vi "SaveRestore_Turret_Homing_Calibration.vi"(2 "ReadWrite_Mode":T1, 3 "Turret_Offset (SensorUnits)":i32) -> (0 "Turret_Home_Set":i32, 1 "Load/Save_successful?":bool)   [LabVIEW 2019]
uses:
  TypeDefs/Read_or_Write.ctl
  <vilib>/Utility/file.llb/Read Delimited Spreadsheet (I64).vi
  <vilib>/Utility/file.llb/Write Delimited Spreadsheet (I64).vi
panel:
  in  "Shooter ID File":path=path "/home/lvuser/turrethome"
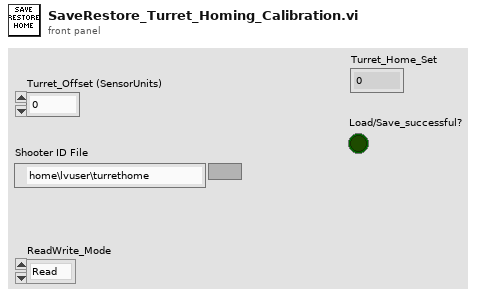
[diagram p1: front panel]
types:
  T1 = typedef "Read_or_Write.ctl" = enum16{"Read", "Write"}
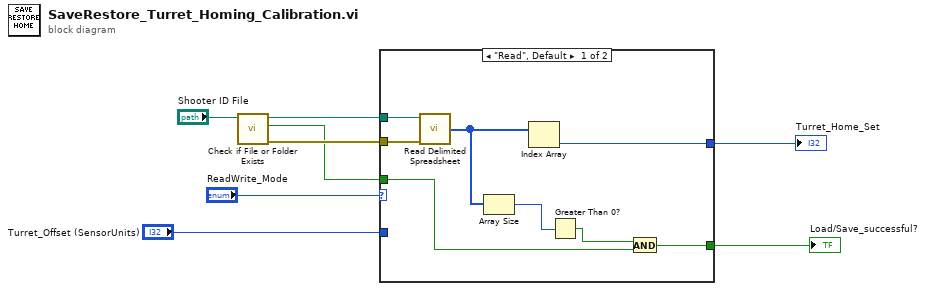
[diagram p0: block diagram]
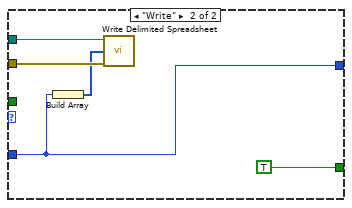
[diagram p2: hidden frame]
diagram:
  n1 = call <vilib>:"Check if File or Folder Exists.vi"("path"="Shooter ID File") -> ("error out"=w4:errorcluster, "file or folder exists?"=w2:bool, "dup path"=w5:path)  [unwired: 8 in]
  n2 = case shown="\"Read\", Default" "ReadWrite_Mode" {
    tunnel: "Turret_Offset (SensorUnits)" -> [_ w19]
    tunnel: [w14 w19] -> w3
    tunnel: w5 -> [w16 w21]
    tunnel: w4 -> [w15 w20]
    tunnel: w2 -> [w13 _]
    tunnel: [w9 TRUE] -> w1
    frame "Read", Default {
      n3 = call-poly <vilib>:"Read Delimited Spreadsheet.vi"("file path (dialog if empty)"=w16, "error in (no error)"=w15) -> ("first row"=w10:i64[])  [unwired: 8 in, 5 out]
      n4 = Array Size(array=w10) -> (size(s)=w11:i32)
      n5 = Index Array(array=w10) -> (element=w14:i64)  [unwired: 1 in]
      n6 = Greater Than 0?(x=w11) -> (x > 0?=w12:bool)
      n7 = And(x=w12, y=w13) -> (x .and. y?=w9:bool)
    }
    frame "Write" {
      n8 = Build Array(w19) -> (w18:i32[])
      n9 = call-poly <vilib>:"Write Delimited Spreadsheet.vi"("file path (dialog if empty)"=w21, "1D data"=w18, "error in (no error)"=w20) -> ()  [unwired: 11 in, 2 out]
    }
  }
  "Turret_Home_Set" <- w3
  "Load/Save_successful?" <- w1
